vi "ExSpectSetSlitPos.vi"() -> ()   [LabVIEW 2010]
panel:
  in  "Slit Number":i16=1 min=1 max=4 step=1
  in  "Position":dbl format="%.2f"
  out "error out":errorcluster
  in  "error in (no error)":errorcluster
  # "ExSpectSetSlitPos.vi\n(Normal Spectrograph via USB/COM port)\nThis VI will set the current position of the selected slit."
  # "NOTES:\nA properly configured spectometer .ini must be present in the LabVIEW folder for spectrograph operation.\n\nConsult the Toolkit documentation for more information on how to configure this file."
  # "um"
  # "1 = Front Entrance\n 2 = Side Entrance\n 3 = Front Exit\n 4 = Side Exit"
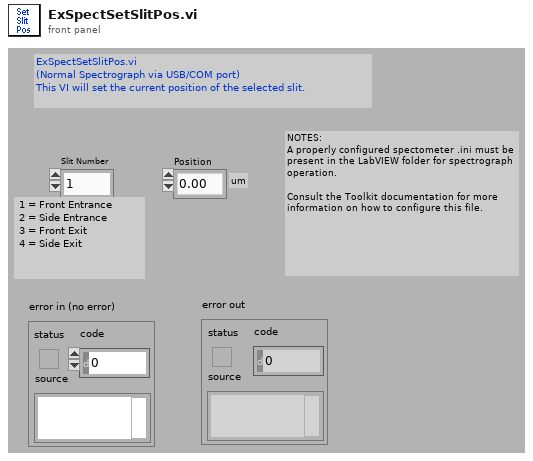
[diagram p1: front panel]
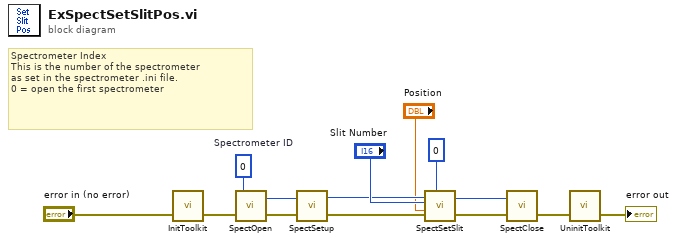
[diagram p0: block diagram]
diagram:
  w12 = u32 0  # Spectrometer ID
  # "Spectrometer Index\nThis is the number of the spectrometer\nas set in the spectrometer .ini file.\n0 = open the first spectrometer"
  n1 = call <userlib>:"InitToolkit.vi"("error in"="error in (no error)") -> ("error out"=w1:errorcluster)
  n2 = call <userlib>:"SpectOpen.vi"("error in"=w1, "Spectrometer ID"=w12) -> ("error out"=w13:errorcluster, "Spectrometer Handle"=w14:u32)  [unwired: 1 in]
  n3 = call <userlib>:"SpectSetup.vi"("error in"=w13, "Spectrometer Handle"=w14) -> ("error out"=w9:errorcluster, "Spectrometer Handle"=w10:u32)
  n4 = call <userlib>:"SpectSetSlit.vi"("Spectrometer Handle"=w10, "Slit Number"="Slit Number", "Position"="Position", "error in"=w9, "Speed"=0) -> ("Spectrometer Handle"=w6:u32, "error out"=w8:errorcluster)
  n5 = call <userlib>:"SpectClose.vi"("error in"=w8, "Spectrometer Handle"=w6) -> ("error out"=w3:errorcluster)
  n6 = call <userlib>:"UninitToolkit.vi"("error in"=w3) -> ("error out"=→"error out":errorcluster)
